vi "Rotate Clockwise.vi"(11 "Motion in":refnum<class "Motion.lvclass">) -> (3 "Motion out":refnum<class "Motion.lvclass">)   [LabVIEW 2021, in "Motion.lvclass"]
uses:
  Motion.lvclass
  Motion.lvclass/Motion.ctl
  Math/Math.lvlib
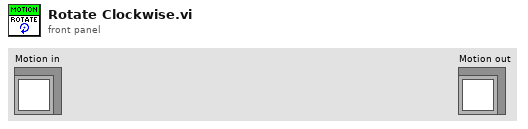
[diagram p1: front panel]
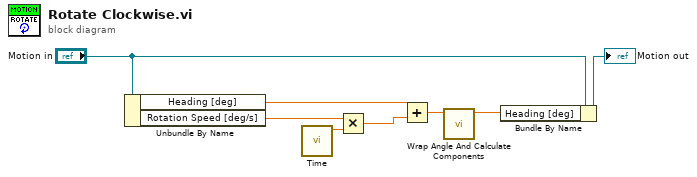
[diagram p0: block diagram]
diagram:
  n1 = Unbundle By Name("Motion in") -> ("Heading [deg]"=w5:sgl, "Rotation Speed [deg/s]"=w2:sgl)
  n2 = call "Time.vi"() -> ("Delta Time [s]"=w3:sgl)  [unwired: 10 in, 1 out]
  n3 = Multiply(x=w2, y=w3) -> (x*y=w1:sgl)
  n4 = Add(x=w5, y=w1) -> (x+y=w4:sgl)
  n5 = call "Wrap Angle And Calculate Components.vi"("Angle in [deg]"=w4) -> ("Angle out [deg]"=w6:sgl)  [unwired: 10 in]
  n6 = Bundle By Name(cluster="Motion in", "Heading [deg]"=w6) -> (→"Motion out":refnum<class "Motion.lvclass">)
